vi "Read FAN2.vi"(8 "error in (no error)":errorcluster, 11 "ParameterConf in":refnum<class "ParameterConf.lvclass">) -> (0 "error out":errorcluster, 1 "Queue Process.Serial Data Gcode":refnum<queue>, 2 "FAN2":dbl min=0.0 max=255.0 step=5.0, 3 "ParameterConf out":refnum<class "ParameterConf.lvclass">)   [LabVIEW 2017, in "ParameterConf.lvclass"]
uses:
  ParameterConf.lvclass
  ParameterConf.lvclass/ParameterConf.ctl
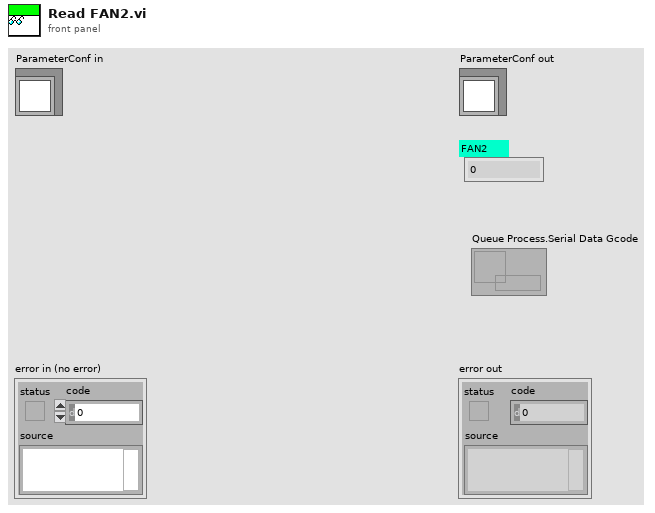
[diagram p1: front panel]
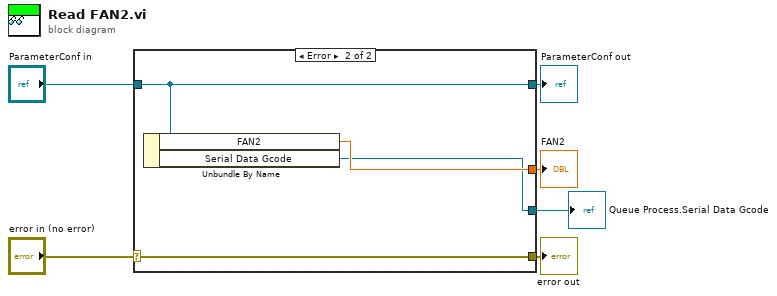
[diagram p0: block diagram]
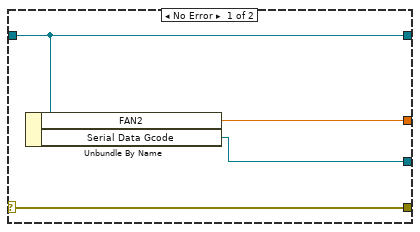
[diagram p2: hidden frame]
diagram:
  n1 = case shown="Error" "error in (no error)" {
    selector: "error in (no error)" -> [w10 w14]
    tunnel: [w10 w14] -> w5
    tunnel: [w9 w13] -> w3
    tunnel: "ParameterConf in" -> [w9 w13]
    tunnel: [w8 w12] -> w2
    tunnel: [w7 w11] -> w1
    frame No Error {
      n2 = Unbundle By Name(w9) -> ("FAN2"=w8:dbl, "Serial Data Gcode"=w7:refnum<queue>)
    }
    frame Error {
      n3 = Unbundle By Name(w13) -> ("FAN2"=w12:dbl, "Serial Data Gcode"=w11:refnum<queue>)
    }
  }
  "error out" <- w5
  "ParameterConf out" <- w3
  "FAN2" <- w2
  "Queue Process.Serial Data Gcode" <- w1
